vi "Set and Get Adaptive Filter Coefficients.vi"() -> ()   [LabVIEW 2019]
doc: "This example demonstrates how to set coefficients to, and get coefficients from, an adaptive filter. This example executes the following steps:\n\n1. Creates an FIR LMS adaptive filter.\n\n2. Sets initial coefficients to this adaptive filter. This step represents a situation in which you have prior knowledge about the coefficients of an unknown system.\n\n3. Creates a second FIR LMS adaptive filter with no initial coefficients. This step represents a situation in which you do not have prior knowledge about the coefficients of an unknown system.\n\n4. Uses each filter to identify the impulse response of an unknown system.\n\n5. Retrieves the coefficients from each filter.\n\n6. Plots the coefficients of each filter alongside the coefficients of the unknown system.\n\nAfter you run the VI, compare the error signals and accuracy of the filter coefficients to the coefficients of the unknown system."
uses:
  <vilib>/addons/Adaptive Filters/Create/AFT Create FIR LMS (Real).vi
  <vilib>/addons/Adaptive Filters/Analysis/AFT Set Coefficients (FIR, Real).vi
  <vilib>/addons/Adaptive Filters/Processing/AFT Filter Signal and Update Coefficients (Real, PtByPt).vi
  <vilib>/addons/Adaptive Filters/Analysis/AFT Get Coefficients (FIR, Real).vi
  <vilib>/addons/Adaptive Filters/NI_AdaptiveFilter.lvlib
panel:
  out "Error Signals":dbl[][](graph)
  in  "Step Size":dbl=0.002 min=0.0 step=0.001
  in  "Filter Length":i32=25 min=2
  out "Coefficients":dbl[][](graph)
  # "Select Help>>Show Context Help and move the cursor over the VI icon of this example for more information."
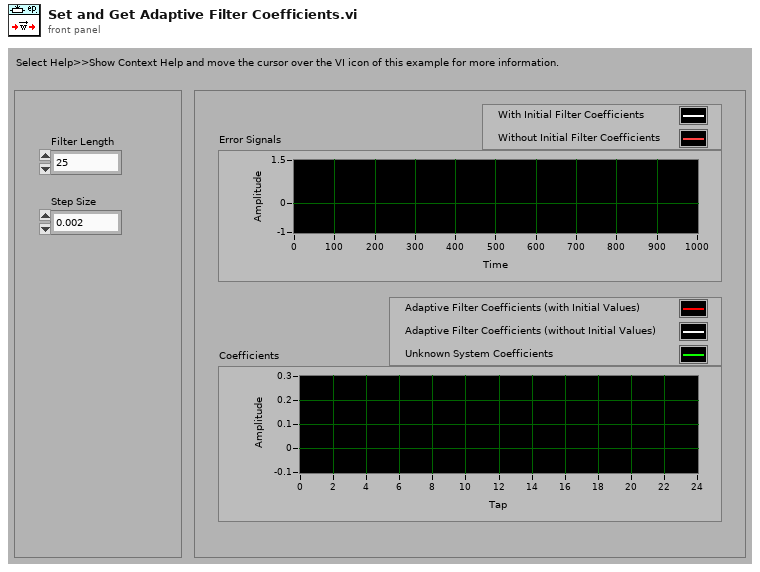
[diagram p1: front panel]
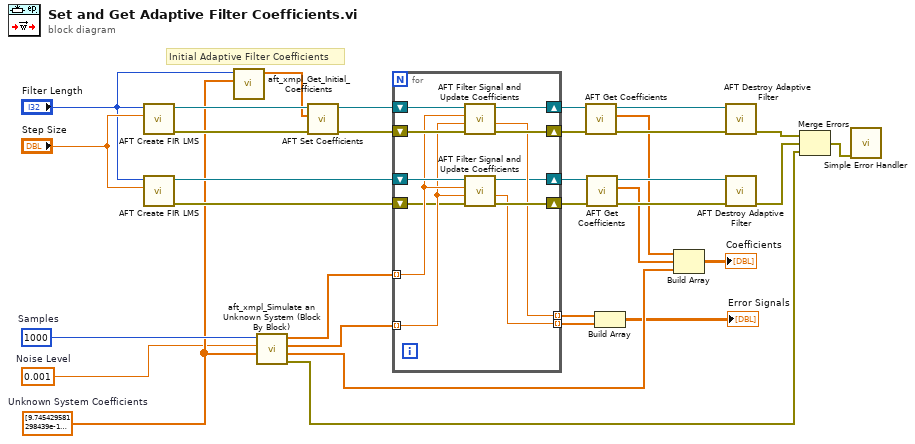
[diagram p0: block diagram]
diagram:
  w6 = 1000  # Samples
  w3 = 0.001  # Noise Level
  w5 = dbl[] [9.745429581298439e-18, 0.020461734458116075, 0.031830988618379075, 0.025008786559919588, -4.508492604200419e-17, -0.03215415414846812, -0.053051647697298455, -0.04501581580785527, 8.042442250270995e-17, 0.07502635967975894, 0.15915494309189543, 0.2250790790392766, 0.25, 0.2250790790392766, 0.15915494309189543, 0.07502635967975894, 8.042442250270995e-17, -0.04501581580785527, -0.053051647697298455, -0.03215415414846812, -4.508492604200419e-17, 0.025008786559919588, 0.031830988618379075, 0.020461734458116075, 9.745429581298439e-18]  # Unknown System Coefficients
  # "Initial Adaptive Filter Coefficients"
  n1 = call-poly <vilib>:"AFT Create FIR LMS.vi"("step size"="Step Size", "filter length"="Filter Length") -> ("error out"=w27:errorcluster, "adaptive filter out"=w28:refnum<k20>)  [unwired: 2 in, 6 out]
  n2 = call-poly <vilib>:"AFT Create FIR LMS.vi"("step size"="Step Size", "filter length"="Filter Length") -> ("error out"=w21:errorcluster, "adaptive filter out"=w23:refnum<k20>)  [unwired: 2 in, 6 out]
  n3 = call "aft_xmpl_Get_Initial_Coefficients.vi"("unknown system coefficients"=w5, "filter length"="Filter Length") -> ("initial coefficients"=w15:dbl[])  [unwired: 9 out]
  n4 = call "aft_xmpl_Simulate an Unknown System (Block By Block).vi"("unknown system coefficients"=w5, "noise level"=w3, "samples"=w6) -> ("error out"=w2:errorcluster, "unknown system coefficients"=w4:dbl[], "response signal"=w7:dbl[], "stimulus signal"=w8:dbl[])  [unwired: 1 in, 4 out]
  n5 = call-poly <vilib>:"AFT Set Coefficients.vi"("error in (no error)"=w27, "coefficients"=w15, "adaptive filter in"=w28) -> ("error out"=w25:errorcluster, "adaptive filter out"=w26:refnum<k20>)  [unwired: 7 out]
  n6 = for {
    shift-right: [w42] -> w33
    shift-left: w26 -> [w44]
    shift-right: [w41] -> w32
    shift-left: w25 -> [w43]
    tunnel: w8 -> [w38] mode=indexing
    tunnel: w7 -> [w37] mode=indexing
    tunnel: [w40] -> w16 mode=indexing
    tunnel: [w34] -> w17 mode=indexing
    shift-right: [w36] -> w22
    shift-left: w23 -> [w39]
    shift-right: [w45] -> w20
    shift-left: w21 -> [w35]
    n7 = call-poly <vilib>:"AFT Filter Signal and Update Coefficients.vi"("error in (no error)"=w43, "d(n)"=w37, "x(n)"=w38, "adaptive filter in"=w44) -> ("error out"=w41:errorcluster, "e(n)"=w40:dbl, "adaptive filter out"=w42:refnum<k20>)  [unwired: 2 in, 3 out]
    n8 = call-poly <vilib>:"AFT Filter Signal and Update Coefficients.vi"("error in (no error)"=w35, "d(n)"=w37, "x(n)"=w38, "adaptive filter in"=w39) -> ("error out"=w45:errorcluster, "e(n)"=w34:dbl, "adaptive filter out"=w36:refnum<k20>)  [unwired: 2 in, 3 out]
  }
  n9 = call-poly <vilib>:"AFT Get Coefficients.vi"("error in (no error)"=w32, "adaptive filter in"=w33) -> ("error out"=w30:errorcluster, "coefficients"=w13:dbl[], "adaptive filter out"=w31:refnum<k20>)  [unwired: 7 out]
  n10 = call-poly <vilib>:"AFT Get Coefficients.vi"("error in (no error)"=w20, "adaptive filter in"=w22) -> ("error out"=w18:errorcluster, "coefficients"=w12:dbl[], "adaptive filter out"=w19:refnum<k20>)  [unwired: 7 out]
  n11 = Build Array(w16, w17) -> (→"Error Signals":dbl[][])
  n12 = Build Array(w13, w12, w4) -> (→"Coefficients":dbl[][])
  n13 = call <vilib>:"AFT Destroy Adaptive Filter.vi"("error in (no error)"=w30, "adaptive filter in"=w31) -> ("error out"=w11:errorcluster)  [unwired: 9 out]
  n14 = call <vilib>:"AFT Destroy Adaptive Filter.vi"("error in (no error)"=w18, "adaptive filter in"=w19) -> ("error out"=w10:errorcluster)  [unwired: 9 out]
  n15 = Merge Errors(w11, w10, w2) -> (w9:errorcluster)
  n16 = call <vilib>:"Simple Error Handler.vi"("error in (no error)"=w9) -> ()  [unwired: 1 in, 8 out]
